vi "twist_msg.vi"(11 "vel_cal":cluster{"rot_z":dbl, "lin_x":dbl}) -> (3 "msg out":string)   [LabVIEW 2014]
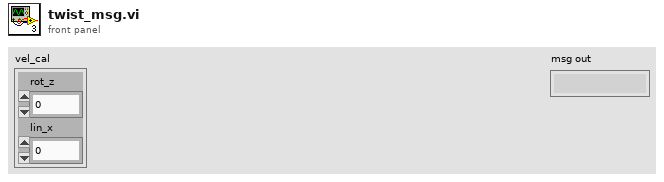
[diagram p1: front panel]
types:
  T1 = cluster{"Linear":cluster{"x":dbl, "y":dbl, "z":dbl}, "Angular":cluster{"x":dbl, "y":dbl, "z":dbl}}
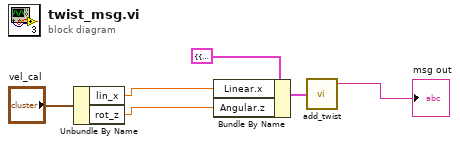
[diagram p0: block diagram]
diagram:
  n1 = Unbundle By Name("vel_cal") -> ("lin_x"=w3:dbl, "rot_z"=w2:dbl)
  n2 = Bundle By Name(cluster=T1 {"Linear"={"x"=0.0, "y"=0.0, "z"=0.0}, "Angular"={"x"=0.0, "y"=0.0, "z"=0.0}} ("Twist"), "Linear.x"=w3, "Angular.z"=w2) -> (w5:T1)
  n3 = call <userlib>:"add_twist.vi"("Twist"=w5) -> ("msg out"=→"msg out":string)  [unwired: 4 in]
